vi "Close & Abort VIs.vi"(8 "Error In":errorcluster, 9 "Abort (T)":bool=TRUE, 11 "VI Paths":path[](array[path])) -> (0 "Error Out":errorcluster)   [LabVIEW 2021, in "Utilities.lvlib"]
uses:
  Utilities.lvlib
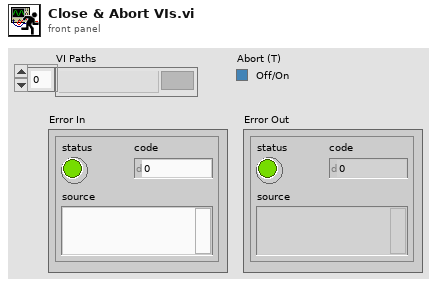
[diagram p1: front panel]
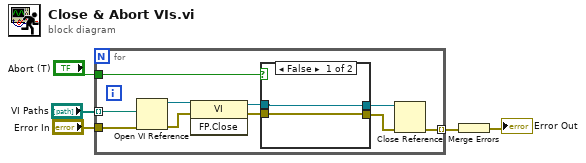
[diagram p0: block diagram]
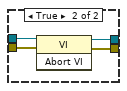
[diagram p2: hidden frame]
diagram:
  n1 = for {
    tunnel: "VI Paths" -> [w15] mode=indexing
    tunnel: "Error In" -> [w9]
    tunnel: [w8] -> w3 mode=indexing
    tunnel: "Abort (T)" -> [w7]
    n2 = Open VI Reference(vi path=w15, error in (no error)=w9) -> (vi reference=w14:refnum<vi>, error out=w13:errorcluster)  [unwired: 4 in]
    n3 = invoke class="VI" method="FP.Close"(reference=w14, error in=w13) -> (reference out=w12:refnum<vi>, error out=w11:errorcluster)  [unwired: 1 in, 1 out]
    n4 = case shown="False" w7 {
      tunnel: w12 -> [w17 w21]
      tunnel: w11 -> [w16 w20]
      tunnel: [w16 w18] -> w10
      tunnel: [w17 w19] -> w6
      frame False {
      }
      frame True {
        n5 = invoke class="VI" method="Abort VI"(reference=w21, error in=w20) -> (reference out=w19:refnum<vi>, error out=w18:errorcluster)  [unwired: 1 in, 1 out]
      }
    }
    n6 = Close Reference(reference=w6, error in (no error)=w10) -> (error out=w8:errorcluster)
  }
  n7 = Merge Errors(w3) -> (→"Error Out":errorcluster)
